vi "Read Compilation Type.vi"(9 "RasPi Compiler in":refnum<class "RasPi Compiler.lvclass">) -> (3 "RasPi Compiler out":refnum<class "RasPi Compiler.lvclass">, 4 "Compilation Type":T1)   [LabVIEW 2014, in "RasPi Compiler.lvclass"]
uses:
  RasPi Compiler.lvclass
  Compile and Download App/Custom Controls/CompileType.ctl
  RasPi Compiler.lvclass/RasPi Compiler.ctl
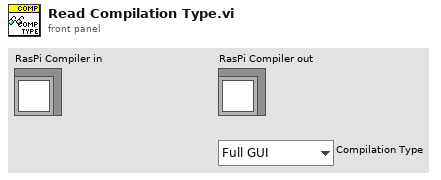
[diagram p1: front panel]
types:
  T1 = typedef "CompileType.ctl" = enum16{"Full GUI", "Console App"}
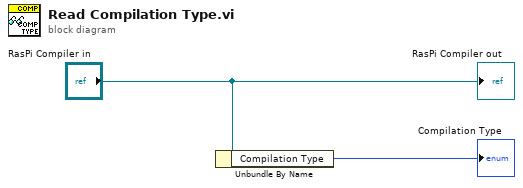
[diagram p0: block diagram]
diagram:
  n1 = Unbundle By Name("RasPi Compiler in") -> ("Compilation Type"=→"Compilation Type":T1)
  "RasPi Compiler out" <- "RasPi Compiler in"
